vi "例5-7.vi"() -> ()   [LabVIEW 2019]
uses:
  <vilib>/DAQmx/write.llb/DAQmx Write (Digital 1D Bool NChan 1Samp 1Line).vi
  <vilib>/DAQmx/create/channels.llb/DAQmx Create Channel (DO-Digital Output).vi
  <vilib>/DAQmx/miscellaneous.llb/DAQmx Fill In Error Info.vi
panel:
  in  "停止":bool
  in  "I/O线输出值":bool[](array[boolean])
  in  "I/O线":tag[](array[tag])
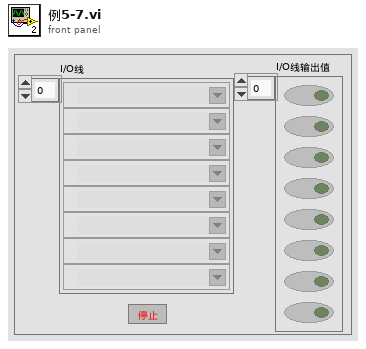
[diagram p1: front panel]
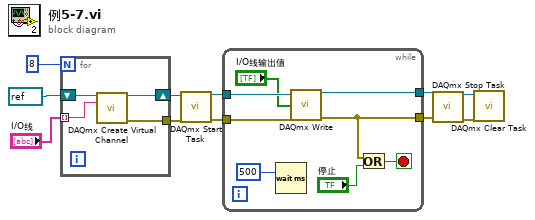
[diagram p0: block diagram]
diagram:
  n1 = for {
    N: 8 -> [_]
    shift-right: [w14] -> w9
    shift-left: refnum<k21> refnum ("task in") -> [w15]
    tunnel: [w13] -> w2
    tunnel: "I/O线" -> [w12] mode=indexing
    n2 = call-poly <vilib>:"DAQmx Create Virtual Channel.vi"("task in"=w15, "lines"=w12) -> ("task out"=w14:refnum<k21>, "error out"=w13:errorcluster)  [unwired: 12 in]
  }
  n3 = call <vilib>:"DAQmx Start Task.vi"("task/channels in"=w9, "error in"=w2) -> ("task out"=w6:refnum<k21>, "error out"=w4:errorcluster)  [unwired: 12 in]
  n4 = while {
    tunnel: w6 -> [w23]
    tunnel: [w22] -> w5
    tunnel: w4 -> [w21]
    tunnel: [w17] -> w3
    stop <- w19 stop-if-true
    n5 = Wait (ms)(milliseconds to wait=500) -> ()  [unwired: 1 out]
    n6 = call-poly <vilib>:"DAQmx Write.vi"("task/channels in"=w23, "data"="I/O线输出值", "error in"=w21) -> ("task out"=w22:refnum<k21>, "error out"=w17:errorcluster)  [unwired: 10 in, 1 out]
    n7 = Or(x=w17, y="停止") -> (x .or. y?=w19:bool)
  }
  n8 = call <vilib>:"DAQmx Stop Task.vi"("task/channels in"=w5, "error in"=w3) -> ("task out"=w8:refnum<k21>, "error out"=w7:errorcluster)  [unwired: 12 in]
  n9 = call <vilib>:"DAQmx Clear Task.vi"("task in"=w8, "error in"=w7) -> ()  [unwired: 13 in, 1 out]
